vi "Process.vi"(8 "error in":errorcluster, 11 "DSP":refnum<class "DSP.lvclass">) -> (0 "error out":errorcluster, 3 "DSP out":refnum<class "DSP.lvclass">)   [LabVIEW 2016, in "DSP.lvclass"]
doc: "---------------------------------------------------------------\nJKI State Machine Objects™\nhttp://jki.net/state-machine-objects/\nCopyright (C) 2005-2015, JKI <info@jki.net>\nALL RIGHTS RESERVED"
uses:
  DSP.lvclass
  C:/Program Files (x86)/National Instruments/LabVIEW 2016/vi.lib/JKI/JKI SMO/SMO/SMO.lvclass
  <vilib>/JKI/JKI SMO/SMO/Typedefs/Parent Call--Enum.ctl
  Typedefs/PrivateEvents--DSP.RunCalculation.ctl
  Typedefs/LP_Config.ctl
  DSP.lockin/Typedefs/Lockin_Config.ctl
  Typedefs/FFT_Config.ctl
  <vilib>/Analysis/4window.llb/windowTd.ctl
  <vilib>/measure/maspectr.llb/Power Spectrum and PSD Export Mode.ctl
  <vilib>/JKI/JKI SMO/SMO/SMO.lvclass
  DSP.lockin/DSP.lockin.lvclass
  <vilib>/Analysis/NI_AALPro.lvlib
  <vilib>/measure/NI_MAPro.lvlib
  DSP.Filter/DSP.Filter.lvclass
panel:
  # "For instructions on how to use the JKI State Machine Objects, examples and video tutorials, visit:\nhttp://jki.net/state-machine-objects/\n\nJKI State Machine Objects™\nhttp://jki.net/state-machine-objects/\nCopyright (C) 2005-2015, JKI <info@jki.net>\nALL RIGHTS RESERVED"
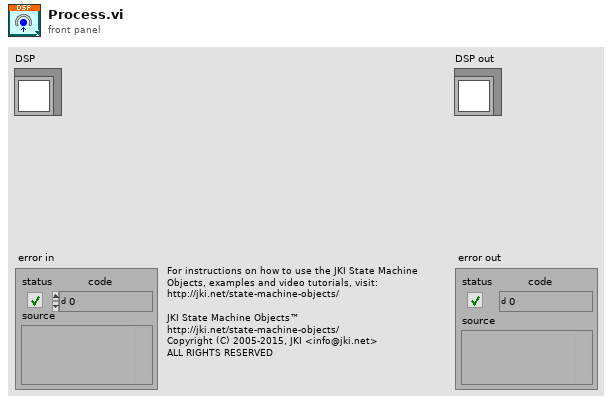
[diagram p1: front panel]
types:
  T1 = typedef "SMO.lvclass/Parent Call--Enum.ctl" = enum16{"Allows parent to run", "Does not request parent to run"}
  T2 = enum32{"invalid app kind", "Development System", "Run Time System", "Student Edition", "Embedded LabVIEW", "Evaluation", "Custom"}
  T3 = typedef "DSP.lvclass/PrivateEvents--DSP.RunCalculation.ctl" = cluster{"RunCalculation":cluster{"adjust gain":bool, "subtract offset":bool, "60 Hz prefilter":bool, "LP prefilter":bool, "lockin":bool, "FFT":bool, "gain":dbl[], "offset":dbl[], "LP config":T4, "Lockin config":T5, "FFT config":T6}}
  T4 = typedef "DSP.lvclass/LP_Config.ctl" = cluster{"high cutoff freq [Hz]":dbl}
  T5 = typedef "DSP.lockin.lvclass/Lockin_Config.ctl" = cluster{" f (Hz)":dbl, "phi (deg)":dbl, "TC (s)":dbl, "order":i32}[]
  T6 = typedef "DSP.lvclass/FFT_Config.ctl" = cluster{"averaging parameters":cluster{"averaging mode":enum16{"No averaging", "Vector averaging", "RMS averaging", "Peak hold"}, "weighting mode":enum16{"Linear", "Exponential"}, "number of averages":u32}, "window":T7, "export mode":T8, "window parameter":dbl, "restart averaging (F)":bool}
  T7 = typedef "NI_AALPro.lvlib/windowTd.ctl" = u32
  T8 = typedef "NI_MAPro.lvlib/Power Spectrum and PSD Export Mode.ctl" = u16
  T9 = enum32{"Invalid", "Standard", "Closed", "Hidden", "Minimized", "Maximized"}
  T10 = enum32{"Bad", "Idle", "Run top level", "Running"}
  T11 = typedef "DSP.lvclass/PrivateEvents--DSP.setWaveform.ctl" = waveform(dbl)[]
  T12 = cluster{"Core":cluster{"Current VI Reference":refnum<vi>, "Close Panel on Exit?":bool, "error":errorcluster}, "Self Reference":refnum<class "DSP.lvclass">, "Your string data":string, "Waveforms":waveform(dbl)[], "RunCalculation":cluster{"adjust gain":bool, "subtract offset":bool, "60 Hz prefilter":bool, "LP prefilter":bool, "lockin":bool, "FFT":bool, "gain":dbl[], "offset":dbl[], "LP config":T4, "Lockin config":T5, "FFT config":T6}}
  T13 = cluster{"adjust gain":bool, "subtract offset":bool, "60 Hz prefilter":bool, "LP prefilter":bool, "lockin":bool, "FFT":bool, "gain":dbl[], "offset":dbl[], "LP config":T4, "Lockin config":T5, "FFT config":T6}
  T14 = cluster{"Current VI Reference":refnum<vi>, "Close Panel on Exit?":bool, "error":errorcluster}
  T15 = typedef "SMO.lvclass/Protected Events.ctl" = cluster{"StopProcesses":refnum<user-event>, "AbortProcesses":refnum<user-event>, "Config Changed":refnum<user-event>, "Dependency":refnum<user-event>}
  T16 = typedef "DSP.lvclass/PrivateEvents--Cluster.ctl" = cluster{"setWaveform":refnum<user-event>, "RunCalculation":refnum<user-event>}
  T17 = typedef "DSP.lockin.lvclass/LockinResults.ctl" = T18[]
  T18 = typedef "DSP.lockin.lvclass/LockinResult.ctl" = cluster{"X":dbl, "Y":dbl, "R":dbl, "Theta":dbl, "AVG":dbl, "f":dbl}
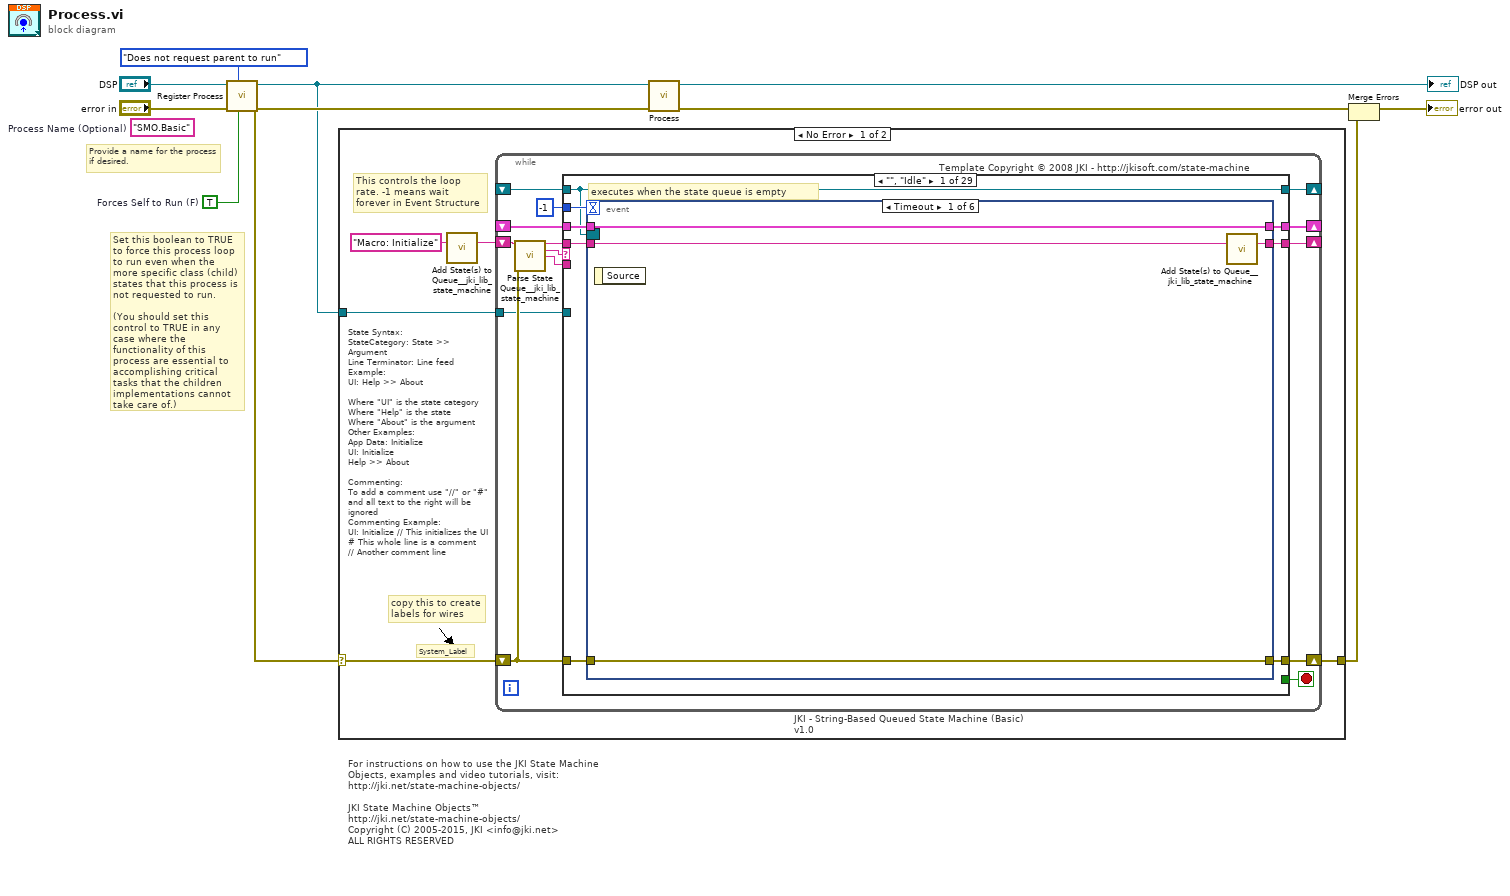
[diagram p0: block diagram]
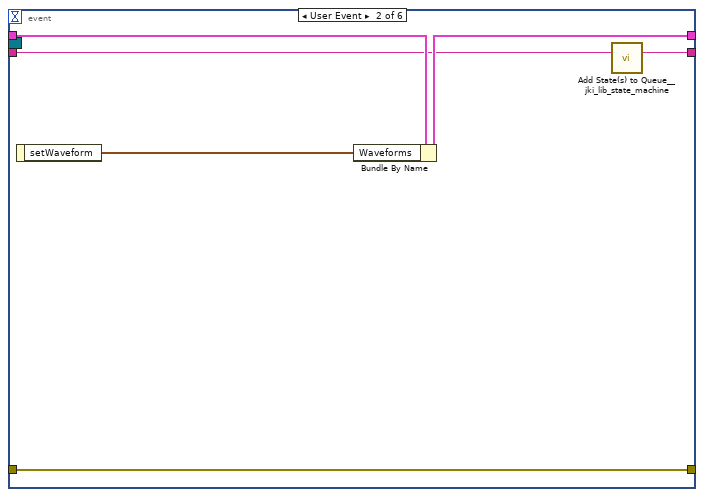
[diagram p2: hidden frame]
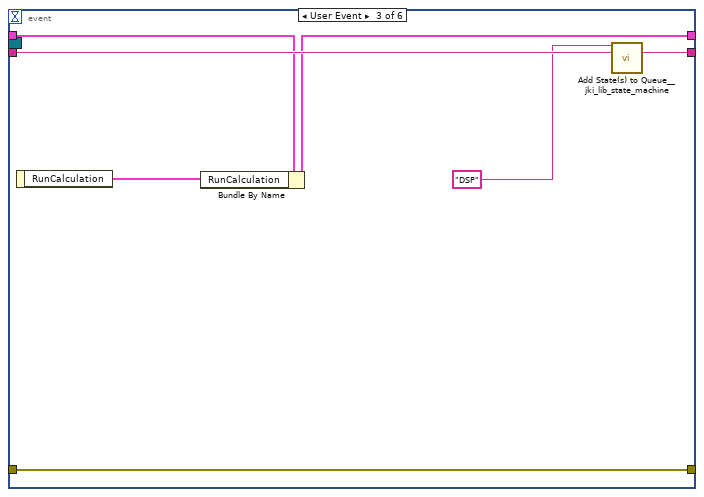
[diagram p3: hidden frame]
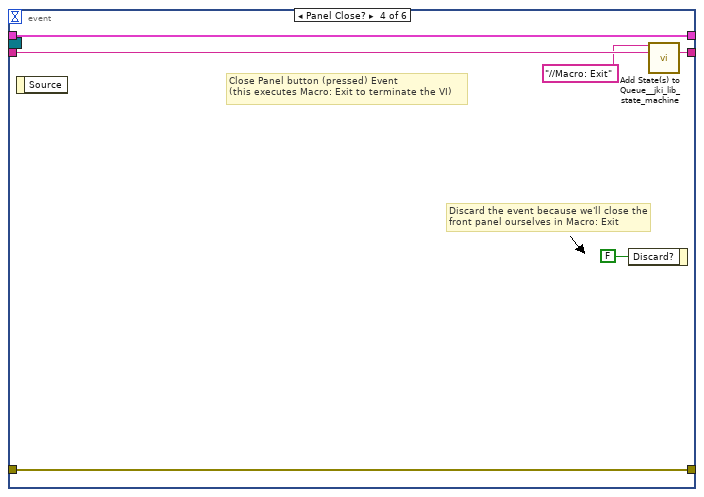
[diagram p4: hidden frame]
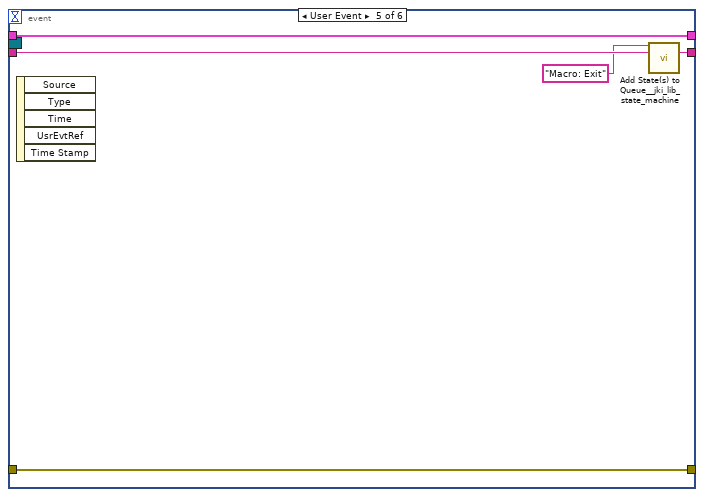
[diagram p5: hidden frame]
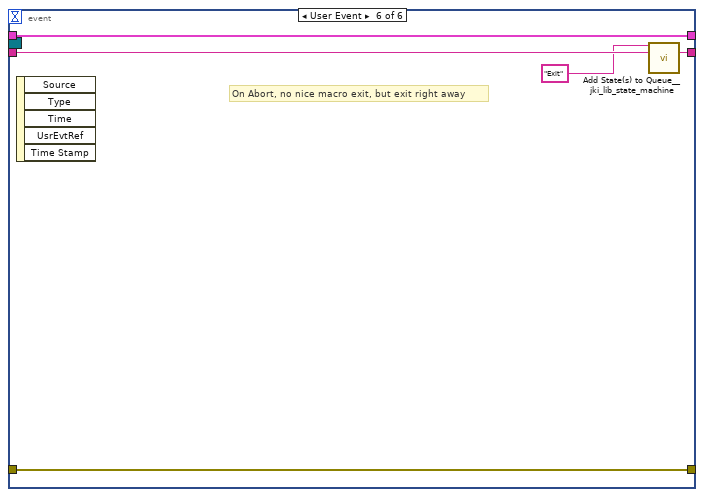
[diagram p6: hidden frame]
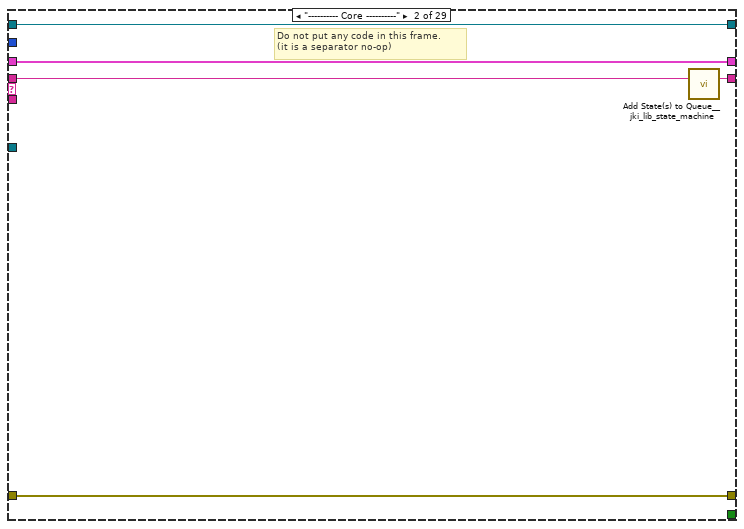
[diagram p7: hidden frame]
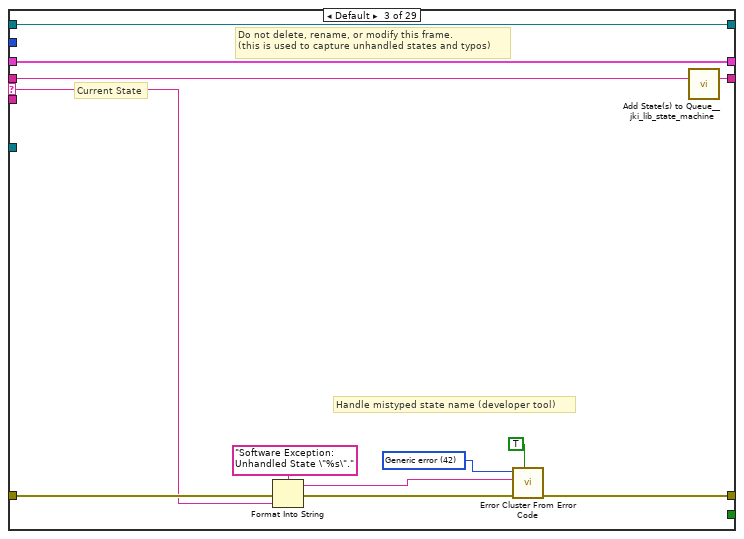
[diagram p8: hidden frame]
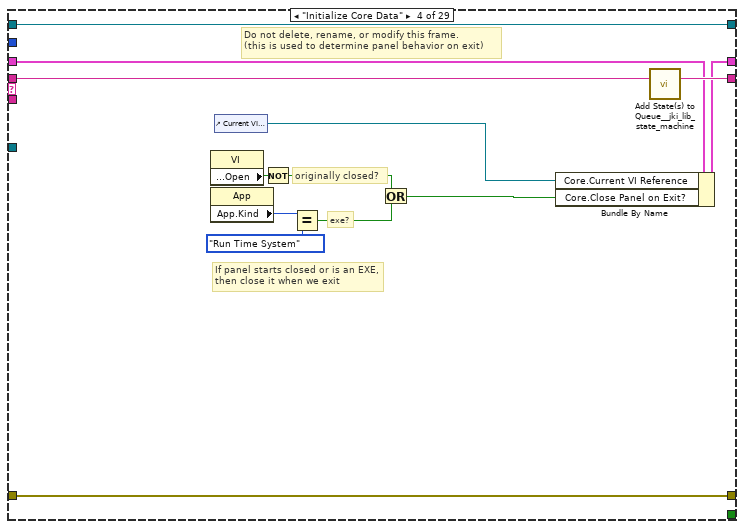
[diagram p9: hidden frame]
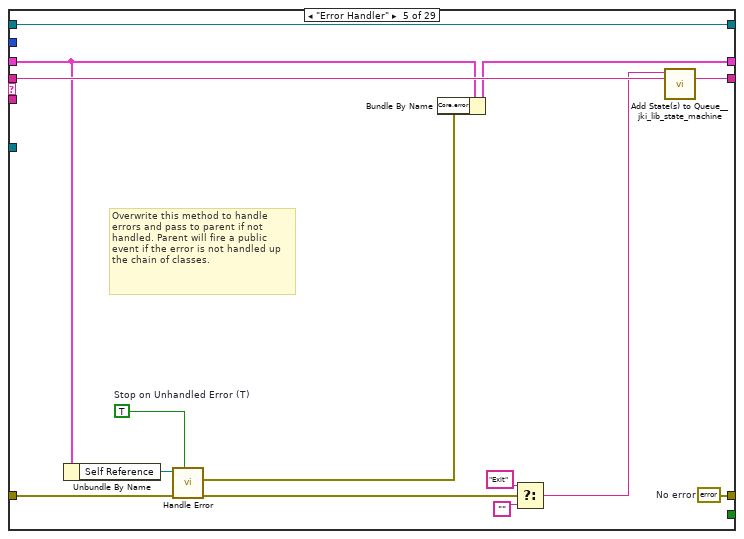
[diagram p10: hidden frame]
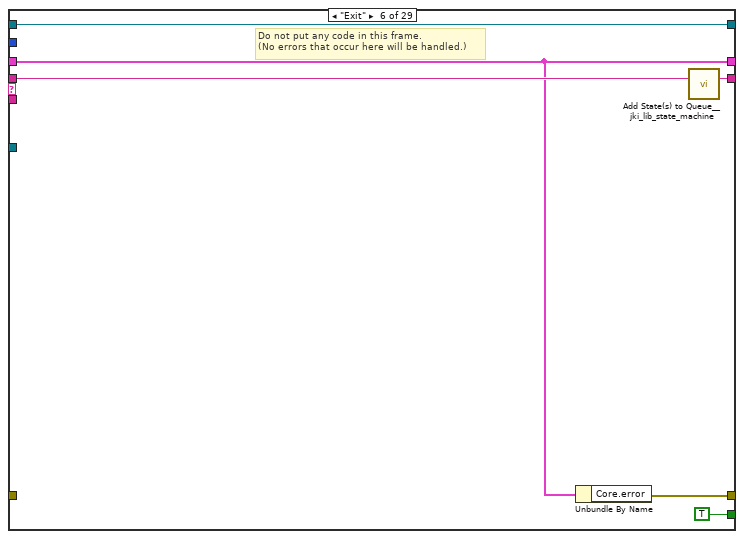
[diagram p11: hidden frame]
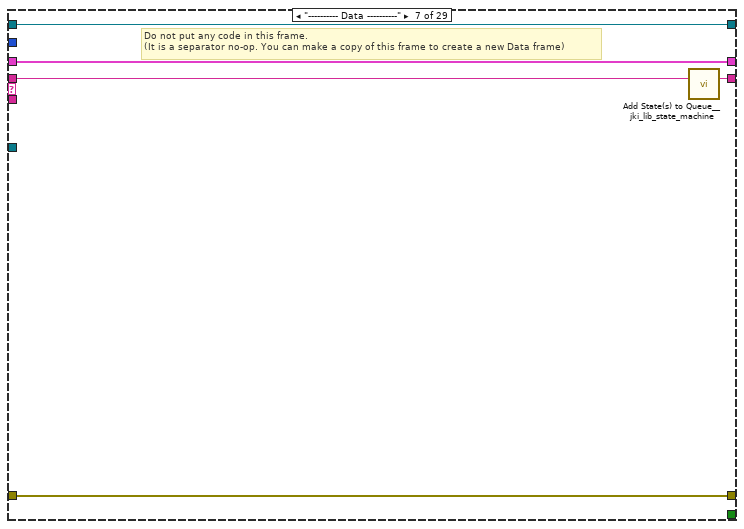
[diagram p12: hidden frame]
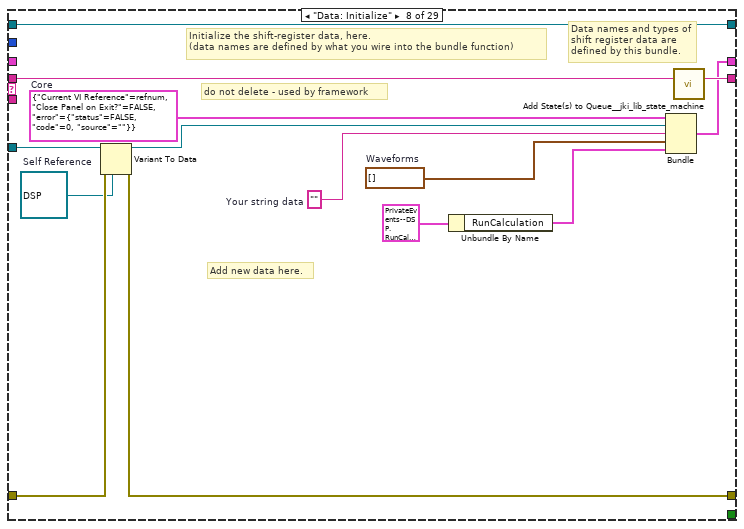
[diagram p13: hidden frame]
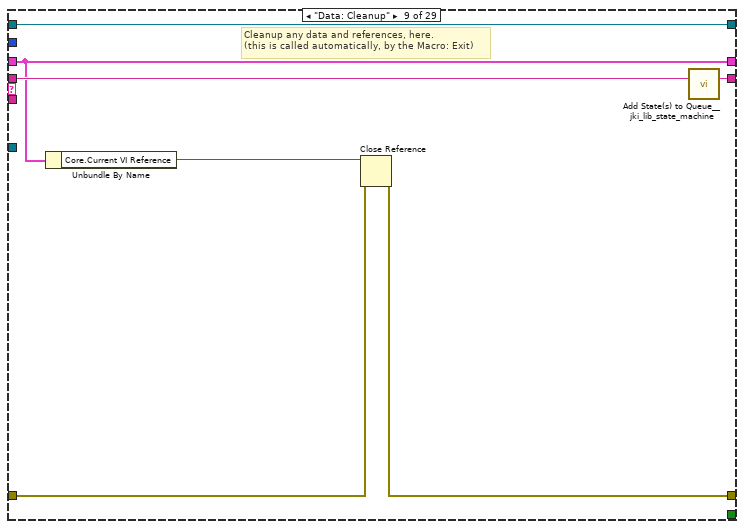
[diagram p14: hidden frame]
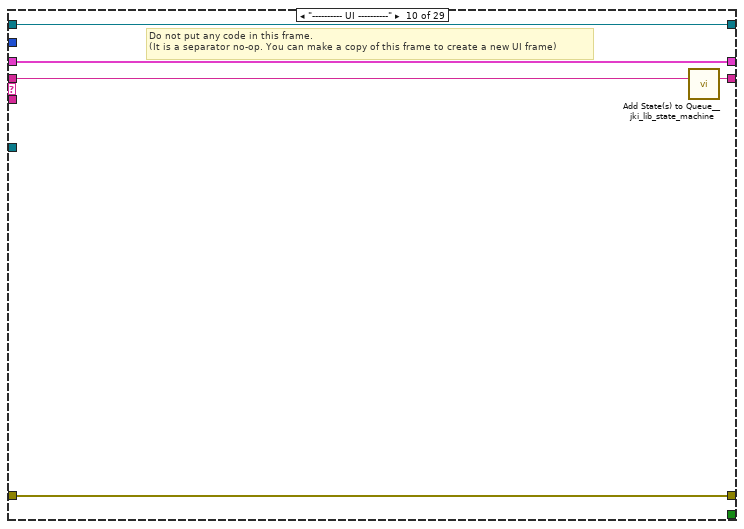
[diagram p15: hidden frame]
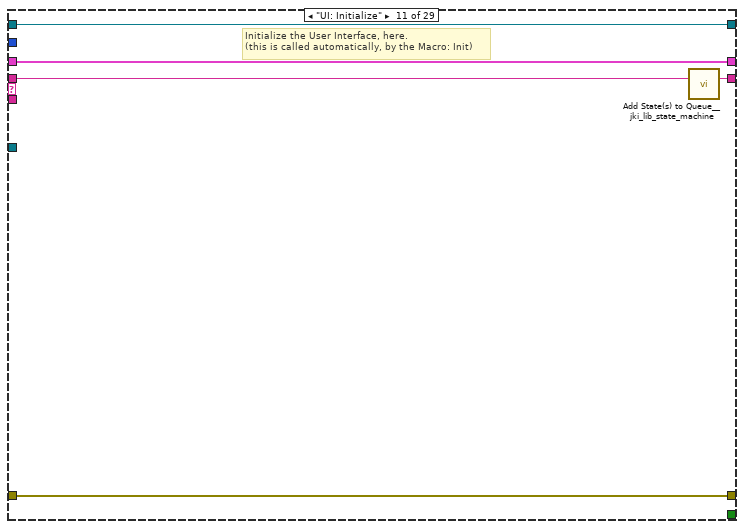
[diagram p16: hidden frame]
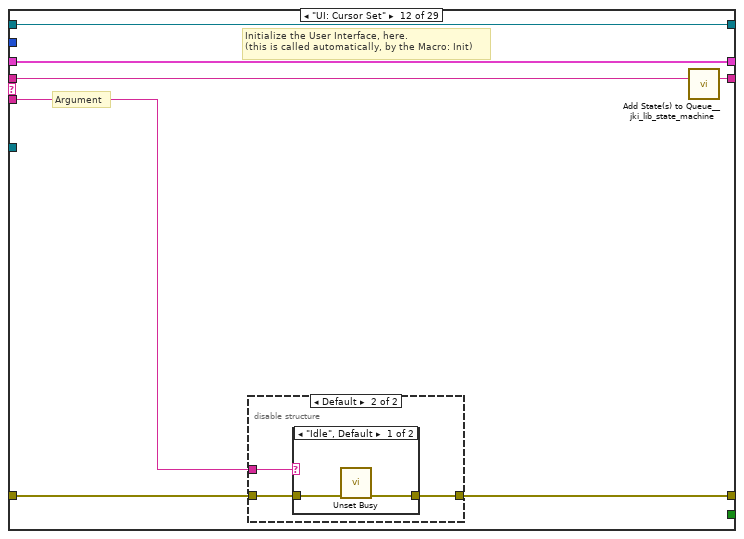
[diagram p17: hidden frame]
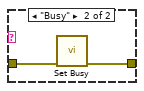
[diagram p19: hidden frame]
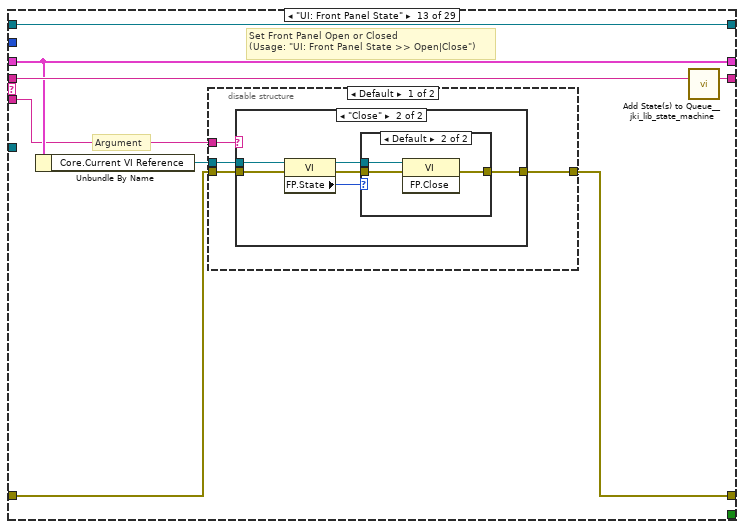
[diagram p20: hidden frame]
diagram:
  w1 = TRUE  # Forces Self to Run (F)
  (unwired) "SMO.Basic"  # Process Name (Optional)
  # "Provide a name for the process\nif desired."
  # "Set this boolean to TRUE to force this process loop to run even when the more specific class (child) states that this process is not requested to run.\n\n(You should set this control to TRUE in any case where the functionality of this process are essential to accomplishing critical tasks that the children implementations cannot take care of.)"
  # "For instructions on how to use the JKI State Machine Objects, examples and video tutorials, visit:\nhttp://jki.net/state-machine-objects/\n\nJKI State Machine Objects™\nhttp://jki.net/state-machine-objects/\nCopyright (C) 2005-2015, JKI <info@jki.net>\nALL RIGHTS RESERVED"
  n1 = call <vilib>:"Register Process.vi"("Forces Self to Run (F)"=w1, "Parent Call"=Parent_Call--Enum."Does not request parent to run", "error in (no error)"="error in", "SMO"="DSP") -> ("error out"=w7:errorcluster, "SMO out"=w6:refnum<class "DSP.lvclass">)  [unwired: 6 in]
  n2 = case shown="No Error" w7 {
    selector: w7 -> [w12 w368]
    tunnel: w6 -> [w13 _]
    tunnel: [w11 w368] -> w3
    frame No Error {
      # "State Syntax:\nStateCategory: State >> Argument\nLine Terminator: Line feed\nExample:\nUI: Help >> About\n\nWhere \"UI\" is the state category\nWhere \"Help\" is the state\nWhere \"About\" is the argument\nOther Examples:\nApp Data: Initialize\nUI: Initialize\nHelp >> About\n\nCommenting:\nTo add a comment use \"//\" or \"#\" and all text to the right will be ignored\nCommenting Example:\nUI: Initialize // This initializes the UI\n# This whole line is a comment\n// Another comment line"
      # "copy this to create labels for wires"
      # "This controls the loop rate. -1 means wait forever in Event Structure"
      # "System_Label"
      n3 = call <vilib>:"Add State(s) to Queue__jki_lib_state_machine.vi"("State(s) in (\"\")"="Macro: Initialize") -> ("States Out"=w15:string)  [unwired: 14 in]
      n4 = while "JKI - String-Based Queued State Machine (Basic) v1.0" {
        shift-right: [w22] -> _
        shift-left: _ -> [w21]
        shift-right: [w25] -> w11
        shift-left: w12 -> [w19]
        shift-right: [w24] -> _
        shift-left: w15 -> [w26]
        tunnel: w13 -> [w18]
        shift-right: [w17] -> _
        shift-left: _ -> [w16]
        stop <- w23 stop-if-true
        # "Template Copyright © 2008 JKI - http://jkisoft.com/state-machine"
        n5 = call <vilib>:"Parse State Queue__jki_lib_state_machine.vi"("State Queue"=w26, "Error In (no error)"=w19) -> ("Remaining States"=w28:string, "Current State"=w29:string, "Arguments"=w27:string)  [unwired: 11 in]
        n6 = case shown="\"\", \"Idle\"" w29 {
          selector: w29 -> [_ _ w77 _ _ _ _ _ _ _ _ _ _ _ _ _ _ _ _ _ _ _ _ _ _ _ _ _ _]
          tunnel: w28 -> [w37 w75 w81 w100 w114 w120 w125 w139 w146 w151 w156 w163 w179 w211 w225 w239 w244 w255 w260 w273 w279 w284 w310 w319 w328 w337 w347 w358 w367]
          tunnel: w27 -> [_ _ _ _ _ _ _ _ _ _ _ w157 w173 _ _ _ _ _ _ _ _ _ _ _ _ _ _ _ _]
          tunnel: w21 -> [w35 w72 w79 w91 w108 w116 w122 _ w141 w148 w154 w161 w175 w208 w221 w230 w241 w252 w257 w271 w277 w282 w306 w315 w324 w334 w344 w355 w363]
          tunnel: [w34 w73 w83 w97 w109 w115 w123 w134 w142 w149 w153 w158 w176 w209 w223 w237 w242 w246 w258 w266 w275 w280 w307 w316 w325 w329 w338 w348 w364] -> w25
          tunnel: w19 -> [w33 w73 w82 w97 w110 _ w123 w135 w143 w149 w153 w159 w177 w209 w223 w237 w242 w247 w258 w267 w275 w280 w307 w316 w325 w330 w339 w354 w364]
          tunnel: [w36 w74 w80 w99 w113 w119 w124 w138 w145 w150 w155 w162 w178 w210 w224 w238 w243 w254 w259 w272 w278 w283 w309 w318 w327 w336 w346 w357 w366] -> w24
          tunnel: [_ _ _ _ _ TRUE _ _ _ _ _ _ _ _ _ _ _ _ _ _ _ _ _ _ _ _ _ _ _] -> w23
          tunnel: [w32 w72 w79 w98 w107 w116 w122 w137 w141 w148 w154 w161 w175 w208 w221 w230 w241 w252 w257 w271 w277 w282 w306 w314 w323 w333 w343 w355 w362] -> w22
          tunnel: -1 ("Timeout") -> [w31 _ _ _ _ _ _ _ _ _ _ _ _ _ _ _ _ _ _ _ _ _ _ _ _ _ _ _ _]
          tunnel: w18 -> [_ _ _ _ _ _ _ w132 _ _ _ _ _ _ _ _ _ _ _ _ _ _ _ _ _ _ _ _ _]
          tunnel: [w30 w71 w76 w88 w112 w117 w121 w130 w140 w147 w152 w160 w172 w207 w222 w231 w240 w253 w256 w270 w276 w281 w308 w317 w326 w335 w345 w356 w365] -> w17
          tunnel: w16 -> [w30 w71 w76 w88 w112 w117 w121 w130 w140 w147 w152 w160 w172 w207 w222 w231 w240 w253 w256 _ w276 w281 w308 w317 w326 w335 w345 w356 w365]
          frame "", "Idle" {
            # "executes when the state queue is empty"
            n7 = event shown="[0] Timeout" {
              selector: w30 -> [_ _ _ _ _ _]
              dyn-events: _ -> [_ _ _ _ _ _]
              timeout: w31 -> [_ _ _ _ _ _]
              tunnel: w37 -> [w41 w43 w53 w60 w65 w70]
              tunnel: [w40 w42 w52 w59 w64 w69] -> w36
              tunnel: w35 -> [w39 w47 w51 w57 w62 w67]
              tunnel: [w38 w44 w54 w58 w63 w68] -> w34
              tunnel: w33 -> [w38 w44 w54 w58 w63 w68]
              tunnel: [w39 w45 w49 w57 w62 w67] -> w32
              event Timeout {
                n8 = event-data() -> ()  [unwired: 1 in, 1 out]
                n9 = call <vilib>:"Add State(s) to Queue__jki_lib_state_machine.vi"("State(s) in (\"\")"=w41) -> ("States Out"=w40:string)  [unwired: 14 in]
              }
              event User Event {
                n10 = event-data() -> ("setWaveform"=w46:T11)  [unwired: 1 in]
                n11 = Bundle By Name(cluster=w47, "Waveforms"=w46) -> (w45:T12)
                n12 = call <vilib>:"Add State(s) to Queue__jki_lib_state_machine.vi"("State(s) in (\"\")"=w43) -> ("States Out"=w42:string)  [unwired: 14 in]
              }
              event User Event {
                n13 = event-data() -> ("RunCalculation"=w50:T13)  [unwired: 1 in]
                n14 = Bundle By Name(cluster=w51, "RunCalculation"=w50) -> (w49:T12)
                n15 = call <vilib>:"Add State(s) to Queue__jki_lib_state_machine.vi"("State(s) in Front (\"\")"="DSP" ("State(s) in Front (\"\")"), "State(s) in (\"\")"=w53) -> ("States Out"=w52:string)  [unwired: 13 in]
              }
              event Panel Close? {
                # "Discard the event because we'll close the front panel ourselves in Macro: Exit"
                # "Close Panel button (pressed) Event\n(this executes Macro: Exit to terminate the VI)"
                n16 = event-data() -> ()  [unwired: 1 in, 1 out]
                n17 = event-data("Discard?"=FALSE) -> ()  [unwired: 1 in, 1 out]
                n18 = call <vilib>:"Add State(s) to Queue__jki_lib_state_machine.vi"("State(s) in Front (\"\")"="//Macro: Exit", "State(s) in (\"\")"=w60) -> ("States Out"=w59:string)  [unwired: 13 in]
              }
              event User Event {
                n19 = event-data() -> ()  [unwired: 1 in, 5 out]
                n20 = call <vilib>:"Add State(s) to Queue__jki_lib_state_machine.vi"("State(s) in Front (\"\")"="Macro: Exit", "State(s) in (\"\")"=w65) -> ("States Out"=w64:string)  [unwired: 13 in]
              }
              event User Event {
                # "On Abort, no nice macro exit, but exit right away"
                n21 = event-data() -> ()  [unwired: 1 in, 5 out]
                n22 = call <vilib>:"Add State(s) to Queue__jki_lib_state_machine.vi"("State(s) in Front (\"\")"="Exit", "State(s) in (\"\")"=w70) -> ("States Out"=w69:string)  [unwired: 13 in]
              }
            }
          }
          frame "---------- Core ----------" {
            # "Do not put any code in this frame.\n(it is a separator no-op)"
            n23 = call <vilib>:"Add State(s) to Queue__jki_lib_state_machine.vi"("State(s) in (\"\")"=w75) -> ("States Out"=w74:string)  [unwired: 14 in]
          }
          frame Default {
            w86 = 42 items=["No error", "Argument error", "Memory is full", "Out of zone", "End of file", "File already open", "Generic file I/O error", "File not found", "File permission error", "Disk is full", "Duplicate path", "Too many files open", "System feature not enabled", "Resource file not found", "Cannot add resource", "Resource not found", "Image not found", "Image memory error", "Pen does not exist", "Config type invalid", "Config token not found", "Config parse error", "Config memory error", "Bad external code format", "Bad external code offset", "External code not present", "Null window", "Destroy window error", "Null menu", "Print aborted", "Bad print record", "Print driver error", "Windows error during printing", "Memory error during printing", "Print dialog error", "Generic print error", "Invalid device refnum", "Device not found", "Device parameter error", "Device unit error", "Cannot open device", "Device call aborted", "Generic error", "Cancelled by user", "Object ID too low", "Object ID too high", "Object not in heap", "Unknown heap", "Unknown object (invalid DefProc)", "Unknown object (DefProc not in table)", "Message out of range", "Invalid (null) method", "Unknown message", "Manager call not supported", "Bad address", "Network operation in progress", "Network operation timed out", "Connection is busy", "Network attribute not supported", "Network error", "Address in use", "System out of memory", "Connection aborted", "Connection refused", "Not connected", "Already connected", "Connection closed", "Initialization error (interapplication manager)", "Bad occurrence", "Wait on unbound occurrence handler", "Occurrence queue overflow", "Datalog type conflict", "Unused", "Unrecognized type (interapplication manager)", "Memory corrupt", "Failed to make temporary DLL", "Old CIN version", "Drag socket not found", "Failed to load drop-object", "Failed to register OLE object", "Failed to release OLE object", "Format specifier type mismatch", "Unknown format specifier", "Too few format specifiers", "Too many format specifiers", "Scan failed", "Newer CIN version", "Error converting to variant", "Runtime menu error", "Password tampered", "Variant attribute not found", "Incompatible variant data type", "Event data is not available", "Event Store is not present", "Occurrence is not found", "Event Queue is not created", "Event info is not available", "Refnum passed is NULL", "Error retrieving Class GUID", "Error retrieving CoClass GUID", "Error retrieving TypeLib GUID.", "Bad built application magic bytes.", "Specific driver is different from the specific driver associated with the Logical Name.", "There is no session opened to the class driver.", "Max Error", "MAX - Error with config objects", "MAX - Error loading configuration", "MAX - Group not supported"]
            # "Current State"
            # "Do not delete, rename, or modify this frame.\n(this is used to capture unhandled states and typos)"
            # "Handle mistyped state name (developer tool)"
            n24 = Format Into String(format string="Software Exception: Unhandled State \"%s\"." ("message"), error in=w82, w77) -> (resulting string=w85:string, error out=w84:errorcluster)  [unwired: 1 in]
            n25 = call <vilib>:"Error Cluster From Error Code.vi"("show call chain? (False)"=TRUE, "error in (no error)"=w84, "error message (\"\")"=w85, "error code (0)"=w86) -> ("error out"=w83:errorcluster)  [unwired: 5 in]
            n26 = call <vilib>:"Add State(s) to Queue__jki_lib_state_machine.vi"("State(s) in (\"\")"=w81) -> ("States Out"=w80:string)  [unwired: 14 in]
          }
          frame "Initialize Core Data" {
            # "Do not delete, rename, or modify this frame.\n(this is used to determine panel behavior on exit)"
            # "originally closed?"
            # "exe?"
            # "If panel starts closed or is an EXE, then close it when we exit"
            n27 = property class="VI"() -> ("Front Panel.Open"=w96:bool)  [unwired: 2 in, 2 out]
            n28 = property class="App"() -> ("App.Kind"=w95:T2)  [unwired: 2 in, 2 out]
            n29 = control-ref of="Current VI Reference"() -> (w89:refnum<vi>)
            n30 = Not(x=w96) -> (.not. x?=w93:bool)
            n31 = Equal?(x=w95, y=T2."Run Time System" ("Application:Kind")) -> (x = y?=w92:bool)
            n32 = Or(x=w93, y=w92) -> (x .or. y?=w90:bool)
            n33 = Bundle By Name(cluster=w91, "Core.Current VI Reference"=w89, "Core.Close Panel on Exit?"=w90) -> (w98:T12)
            n34 = call <vilib>:"Add State(s) to Queue__jki_lib_state_machine.vi"("State(s) in (\"\")"=w100) -> ("States Out"=w99:string)  [unwired: 14 in]
          }
          frame "Error Handler" {
            w101 = TRUE  # Stop on Unhandled Error (T)
            w109 = errorcluster {"status"=FALSE, "code"=0, "source"=""}  # No error
            # "Overwrite this method to handle errors and pass to parent if not handled. Parent will fire a public event if the error is not handled up the chain of classes."
            n35 = Unbundle By Name(w108) -> ("Self Reference"=w111:refnum<class "DSP.lvclass">)
            n36 = call-dynamic "Handle Error.vi"("Stop on Unhandled Error (T)"=w101, "error in"=w110, "SMO"=w111) -> ("handling error"=w102:errorcluster, "Unhandled error"=w105:errorcluster)  [unwired: 6 in, 1 out]
            n37 = Bundle By Name(cluster=w108, "Core.error"=w105) -> (w107:T12)
            n38 = Select(t="Exit", s=w102, f="") -> (s? t:f=w106:string)
            n39 = call <vilib>:"Add State(s) to Queue__jki_lib_state_machine.vi"("State(s) in Front (\"\")"=w106, "State(s) in (\"\")"=w114) -> ("States Out"=w113:string)  [unwired: 13 in]
          }
          frame "Exit" {
            # "Do not put any code in this frame.\n(No errors that occur here will be handled.)"
            n40 = Unbundle By Name(w116) -> ("Core.error"=w115:errorcluster)
            n41 = call <vilib>:"Add State(s) to Queue__jki_lib_state_machine.vi"("State(s) in (\"\")"=w120) -> ("States Out"=w119:string)  [unwired: 14 in]
          }
          frame "---------- Data ----------" {
            # "Do not put any code in this frame.\n(It is a separator no-op. You can make a copy of this frame to create a new Data frame)"
            n42 = call <vilib>:"Add State(s) to Queue__jki_lib_state_machine.vi"("State(s) in (\"\")"=w125) -> ("States Out"=w124:string)  [unwired: 14 in]
          }
          frame "Data: Initialize" {
            w128 = waveform(dbl)[] []  # Waveforms
            w129 = T14 {"Current VI Reference"=refnum, "Close Panel on Exit?"=FALSE, "error"={"status"=FALSE, "code"=0, "source"=""}}  # Core
            w133 = refnum<class "DSP.lvclass"> refnum  # Self Reference
            w136 = ""  # Your string data
            # "do not delete - used by framework"
            # "Add new data here."
            # "Data names and types of shift register data are defined by this bundle."
            # "Initialize the shift-register data, here.\n(data names are defined by what you wire into the bundle function)"
            n43 = Variant To Data(error in=w135, type=w133, Variant=w132) -> (data=w131:refnum<class "DSP.lvclass">, error out=w134:errorcluster)
            n44 = Unbundle By Name(T3 {"RunCalculation"={"adjust gain"=FALSE, "subtract offset"=FALSE, "60 Hz prefilter"=FALSE, "LP prefilter"=FALSE, "lockin"=FALSE, "FFT"=FALSE, "gain"=[], "offset"=[], "LP config"={"high cutoff freq [Hz]"=0.45}, "Lockin config"=[], "FFT config"={"averaging parameters"={"averaging mode"=enum."RMS averaging", "weighting mode"=enum."Exponential", "number of averages"=10}, "window"=1, "export mode"=0, "window parameter"=nan, "restart averaging (F)"=FALSE}}} ("RunCalculation")) -> ("RunCalculation"=w126:T13)
            n45 = Bundle("Core"=w129, "Self Reference"=w131, "Your string data"=w136, "Waveforms"=w128, "RunCalculation"=w126) -> (w137:T12)  [unwired: 1 in]
            n46 = call <vilib>:"Add State(s) to Queue__jki_lib_state_machine.vi"("State(s) in (\"\")"=w139) -> ("States Out"=w138:string)  [unwired: 14 in]
          }
          frame "Data: Cleanup" {
            # "Cleanup any data and references, here.\n(this is called automatically, by the Macro: Exit)"
            n47 = Unbundle By Name(w141) -> ("Core.Current VI Reference"=w144:refnum<vi>)
            n48 = Close Reference(reference=w144, error in (no error)=w143) -> (error out=w142:errorcluster)
            n49 = call <vilib>:"Add State(s) to Queue__jki_lib_state_machine.vi"("State(s) in (\"\")"=w146) -> ("States Out"=w145:string)  [unwired: 14 in]
          }
          frame "---------- UI ----------" {
            # "Do not put any code in this frame.\n(It is a separator no-op. You can make a copy of this frame to create a new UI frame)"
            n50 = call <vilib>:"Add State(s) to Queue__jki_lib_state_machine.vi"("State(s) in (\"\")"=w151) -> ("States Out"=w150:string)  [unwired: 14 in]
          }
          frame "UI: Initialize" {
            # "Initialize the User Interface, here.\n(this is called automatically, by the Macro: Init)"
            n51 = call <vilib>:"Add State(s) to Queue__jki_lib_state_machine.vi"("State(s) in (\"\")"=w156) -> ("States Out"=w155:string)  [unwired: 14 in]
          }
          frame "UI: Cursor Set" {
            # "Argument"
            # "Initialize the User Interface, here.\n(this is called automatically, by the Macro: Init)"
            n52 = disable-structure shown="Default" {
              disable-tunnel: w159 -> [w164 w167]
              disable-tunnel: [w164 w166] -> w158
              disable-tunnel: w157 -> [_ w165]
              frame condition #0 {
              }
              frame condition #1 (active) {
                n53 = case shown="\"Idle\", Default" w165 {
                  tunnel: w167 -> [w169 w171]
                  tunnel: [w168 w170] -> w166
                  frame "Idle", Default {
                    n54 = call <vilib>:"Unset Busy.vi"("error in (no error)"=w169) -> ("error out"=w168:errorcluster)  [unwired: 10 in]
                  }
                  frame "Busy" {
                    n55 = call <vilib>:"Set Busy.vi"("error in (no error)"=w171) -> ("error out"=w170:errorcluster)  [unwired: 9 in, 1 out]
                  }
                }
              }
            }
            n56 = call <vilib>:"Add State(s) to Queue__jki_lib_state_machine.vi"("State(s) in (\"\")"=w163) -> ("States Out"=w162:string)  [unwired: 14 in]
          }
          frame "UI: Front Panel State" {
            # "Argument"
            # "Set Front Panel Open or Closed\n(Usage: \"UI: Front Panel State >> Open|Close\")"
            n57 = Unbundle By Name(w175) -> ("Core.Current VI Reference"=w174:refnum<vi>)
            n58 = disable-structure shown="Default" {
              disable-tunnel: w177 -> [w183 w206]
              disable-tunnel: [w182 w206] -> w176
              disable-tunnel: w174 -> [w181 _]
              disable-tunnel: w173 -> [w180 _]
              frame condition #0 (active) {
                n59 = case shown="\"Close\"" w180 {
                  tunnel: w183 -> [w187 w200]
                  tunnel: [w189 w201] -> w182
                  tunnel: w181 -> [w188 w198]
                  frame "Open", Default {
                    n60 = property class="VI"(reference=w188, error in=w187) -> (reference out=w185:refnum<vi>, error out=w186:errorcluster, "FP.State"=w184:T9)
                    n61 = case shown="\"Closed\"" w184 {
                      tunnel: [w192 w195] -> w189
                      tunnel: w186 -> [w191 w195]
                      tunnel: w185 -> [w190 _]
                      frame "Closed" {
                        n62 = invoke class="VI" method="FP.Open"(reference=w190, error in=w191, "Activate"=TRUE, "State"=T9."Standard") -> (error out=w192:errorcluster)  [unwired: 1 in, 4 out]
                      }
                      frame Default {
                      }
                    }
                  }
                  frame "Close" {
                    n63 = property class="VI"(reference=w198, error in=w200) -> (reference out=w197:refnum<vi>, error out=w199:errorcluster, "FP.State"=w196:T9)
                    n64 = case shown="Default" w196 {
                      tunnel: [w202 w205] -> w201
                      tunnel: w199 -> [w202 w204]
                      tunnel: w197 -> [_ w203]
                      frame "Invalid", "Closed" {
                      }
                      frame Default {
                        n65 = invoke class="VI" method="FP.Close"(reference=w203, error in=w204) -> (error out=w205:errorcluster)  [unwired: 1 in, 2 out]
                      }
                    }
                  }
                }
              }
              frame condition #1 {
              }
            }
            n66 = call <vilib>:"Add State(s) to Queue__jki_lib_state_machine.vi"("State(s) in (\"\")"=w179) -> ("States Out"=w178:string)  [unwired: 14 in]
          }
          frame "---------- Macro ----------" {
            # "Do not put any code in this frame.\n(It is a separator no-op. You can make a copy of this frame to create a new Macro frame)"
            n67 = call <vilib>:"Add State(s) to Queue__jki_lib_state_machine.vi"("State(s) in (\"\")"=w211) -> ("States Out"=w210:string)  [unwired: 14 in]
          }
          frame "Macro: Initialize" {
            w216 = "//UI: Initialize\n//UI: Front Panel State >> Open"  # //UI: Initialize //UI: Front Panel State >> Open
            w212 = "Process: Sync"
            # "Initialization Macro\n(This is called once, when the VI starts)"
            n68 = control-ref of="This VI"() -> (w214:refnum<vi>)
            n69 = property class="VI"(reference=w214) -> ("Exec.State"=w213:T10)  [unwired: 1 in, 2 out]
            n70 = Equal?(x=w213, y=T10."Run top level") -> (x = y?=w219:bool)
            n71 = Select(t=w212, s=w219, f="") -> ()  [unwired: 1 out]
            n72 = call <vilib>:"Add State(s) to Queue__jki_lib_state_machine.vi"("State(s) in Front (\"\")"="Data: Initialize\nInitialize Core Data\nEvents: Register", "State(s) in (\"\")"=w212, "State(s) at Back (\"\")"=w216) -> ("States Out"=w215:string)  [unwired: 12 in]
            n73 = call <vilib>:"Add State(s) to Queue__jki_lib_state_machine.vi"("State(s) in Front (\"\")"=w215, "State(s) in (\"\")"=w225) -> ("States Out"=w224:string)  [unwired: 13 in]
          }
          frame "Macro: Exit" {
            # "Exit Macro\n(This is called once, when the VI exits)"
            n74 = Unbundle By Name(w230) -> ("Core.Close Panel on Exit?"=w236:bool)
            n75 = Select(t="UI: Front Panel State >> Close", s=w236, f="") -> (s? t:f=w233:string)
            n76 = call <vilib>:"Add State(s) to Queue__jki_lib_state_machine.vi"("State(s) in Front (\"\")"="Data: Cleanup\nEvents: Unregister", "State(s) in (\"\")"="Process: Sync", "State(s) at Back (\"\")"="Exit") -> ("States Out"=w227:string)  [unwired: 12 in]
            n77 = call <vilib>:"Add State(s) to Queue__jki_lib_state_machine.vi"("State(s) in (\"\")"=w233, "State(s) at Back (\"\")"=w227) -> ("States Out"=w232:string)  [unwired: 13 in]
            n78 = call <vilib>:"Add State(s) to Queue__jki_lib_state_machine.vi"("State(s) in Front (\"\")"=w232, "State(s) in (\"\")"=w239) -> ("States Out"=w238:string)  [unwired: 13 in]
          }
          frame "---------- Process ----------" {
            # "Template Separator\n(You can make a copy of, or modify, this frame)"
            n79 = call <vilib>:"Add State(s) to Queue__jki_lib_state_machine.vi"("State(s) in (\"\")"=w244) -> ("States Out"=w243:string)  [unwired: 14 in]
          }
          frame "Process: Sync" {
            n80 = Unbundle By Name(w252) -> ("Self Reference"=w248:refnum<class "DSP.lvclass">)
            n81 = call <vilib>:"WaitOnProcessSync.vi"("error in (no error)"=w247, "SMO"=w248) -> ("error out"=w246:errorcluster, "Don't run?"=w251:bool)  [unwired: 7 in, 1 out]
            n82 = Select(t="Data: Cleanup\nEvents: Unregister\nExit", s=w251, f="") -> (s? t:f=w245:string)
            n83 = call <vilib>:"Add State(s) to Queue__jki_lib_state_machine.vi"("State(s) in Front (\"\")"=w245, "State(s) in (\"\")"=w255) -> ("States Out"=w254:string)  [unwired: 13 in]
          }
          frame "---------- Events ----------" {
            # "Template Separator\n(You can make a copy of, or modify, this frame)"
            n84 = call <vilib>:"Add State(s) to Queue__jki_lib_state_machine.vi"("State(s) in (\"\")"=w260) -> ("States Out"=w259:string)  [unwired: 14 in]
          }
          frame "Events: Register" {
            # "Expand to add\nmore events"
            n85 = Unbundle By Name(w271) -> ("Self Reference"=w268:refnum<class "DSP.lvclass">)
            n86 = call <vilib>:"GetProtectedEvents.vi"("SMO"=w268) -> ("error out"=w262:errorcluster, "SMO Protected Events"=w269:T15, "SMO out"=w264:refnum<class "DSP.lvclass">)  [unwired: 8 in]
            n87 = call "DSP.GetPrivateEvents.vi"("error in (no error)"=w262, "DSP"=w264) -> ("error out"=w261:errorcluster, "Private Events"=w263:T16)  [unwired: 7 in, 1 out]
            n88 = register-events(w269, w263) -> (reference out=w270:refnum<event-registration>, error out=w265:errorcluster)  [unwired: 2 in]
            n89 = Merge Errors(w267, w265, w261) -> (w266:errorcluster)
            n90 = call <vilib>:"Add State(s) to Queue__jki_lib_state_machine.vi"("State(s) in (\"\")"=w273) -> ("States Out"=w272:string)  [unwired: 14 in]
          }
          frame "Events: Unregister" {
            n91 = Unregister For Events(event registration refnum=w276, error in=w275) -> (error out=w274:errorcluster)
            n92 = call <vilib>:"Clear Errors.vi"("error in (no error)"=w274) -> ()  [unwired: 5 in, 2 out]
            n93 = call <vilib>:"Add State(s) to Queue__jki_lib_state_machine.vi"("State(s) in (\"\")"=w279) -> ("States Out"=w278:string)  [unwired: 14 in]
          }
          frame "---------- Action ----------" {
            n94 = call <vilib>:"Add State(s) to Queue__jki_lib_state_machine.vi"("State(s) in (\"\")"=w284) -> ("States Out"=w283:string)  [unwired: 14 in]
          }
          frame "DSP" {
            w286 = "\n"
            w293 = "" ("f")
            # "decision tree queues other states"
            n95 = Unbundle By Name(w306) -> ("RunCalculation.adjust gain"=w305:bool, "RunCalculation.subtract offset"=w304:bool, "RunCalculation.60 Hz prefilter"=w303:bool, "RunCalculation.LP prefilter"=w302:bool, "RunCalculation.lockin"=w301:bool, "RunCalculation.FFT"=w300:bool)
            n96 = Select(t="DSP: Gain" ("State(s) in Front (\"\")"), s=w305, f=w293) -> (s? t:f=w292:string)
            n97 = Select(t="DSP: Offset" ("State(s) in Front (\"\")"), s=w304, f=w293) -> (s? t:f=w291:string)
            n98 = Select(t="DSP: 60Hz Filter" ("State(s) in Front (\"\")"), s=w303, f=w293) -> (s? t:f=w290:string)
            n99 = Select(t="DSP: LP Filter" ("State(s) in Front (\"\")"), s=w302, f=w293) -> (s? t:f=w289:string)
            n100 = Select(t="DSP: Lockin" ("State(s) in Front (\"\")"), s=w301, f=w293) -> (s? t:f=w288:string)
            n101 = Select(t="DSP: FFT" ("State(s) in Front (\"\")"), s=w300, f=w293) -> (s? t:f=w285:string)
            n102 = Concatenate Strings(w292, w286, w291, w286, w290, w286, w289, w286, w288, w286, w285) -> (w287:string)
            n103 = call <vilib>:"Add State(s) to Queue__jki_lib_state_machine.vi"("State(s) in Front (\"\")"=w287, "State(s) in (\"\")"=w310) -> ("States Out"=w309:string)  [unwired: 13 in]
          }
          frame "DSP: Gain" {
            # "Divide by amplifier gain"
            n104 = Unbundle By Name(w315) -> ("Waveforms"=w312:waveform(dbl)[], "RunCalculation.gain"=w313:dbl[])
            n105 = Divide(x=w312, y=w313) -> (x/y=w311:waveform(dbl)[])
            n106 = Bundle By Name(cluster=w315, "Waveforms"=w311) -> (w314:T12)
            n107 = call <vilib>:"Add State(s) to Queue__jki_lib_state_machine.vi"("State(s) in (\"\")"=w319) -> ("States Out"=w318:string)  [unwired: 14 in]
          }
          frame "DSP: Offset" {
            # "subtract any instrumental offsets"
            n108 = Unbundle By Name(w324) -> ("Waveforms"=w321:waveform(dbl)[], "RunCalculation.offset"=w322:dbl[])
            n109 = Subtract(x=w321, y=w322) -> (x-y=w320:waveform(dbl)[])
            n110 = Bundle By Name(cluster=w324, "Waveforms"=w320) -> (w323:T12)
            n111 = call <vilib>:"Add State(s) to Queue__jki_lib_state_machine.vi"("State(s) in (\"\")"=w328) -> ("States Out"=w327:string)  [unwired: 14 in]
          }
          frame "DSP: 60Hz Filter" {
            n112 = Unbundle By Name(w334) -> ("Waveforms"=w332:waveform(dbl)[])
            n113 = call "Prefilter_60Hz_Notch.vi"("error in (no error)"=w330, "Waveform In"=w332) -> ("error out"=w329:errorcluster, "Waveform Out"=w331:waveform(dbl)[])  [unwired: 8 in]
            n114 = Bundle By Name(cluster=w334, "Waveforms"=w331) -> (w333:T12)
            n115 = call <vilib>:"Add State(s) to Queue__jki_lib_state_machine.vi"("State(s) in (\"\")"=w337) -> ("States Out"=w336:string)  [unwired: 14 in]
          }
          frame "DSP: LP Filter" {
            n116 = Unbundle By Name(w344) -> ("Waveforms"=w342:waveform(dbl)[], "RunCalculation.LP config.high cutoff freq [Hz]"=w340:dbl)
            n117 = call "Prefilter_LP.vi"("error in (no error)"=w339, "high cutoff freq [Hz]"=w340, "Waveforms In"=w342) -> ("error out"=w338:errorcluster, "Waveforms Out"=w341:waveform(dbl)[])  [unwired: 7 in]
            n118 = Bundle By Name(cluster=w344, "Waveforms"=w341) -> (w343:T12)
            n119 = call <vilib>:"Add State(s) to Queue__jki_lib_state_machine.vi"("State(s) in (\"\")"=w347) -> ("States Out"=w346:string)  [unwired: 14 in]
          }
          frame "DSP: Lockin" {
            n120 = Unbundle By Name(w355) -> ("Self Reference"=w349:refnum<class "DSP.lvclass">, "RunCalculation.Lockin config"=w352:T5, "Waveforms"=w353:waveform(dbl)[])
            n121 = call "Lockin Engine.vi"("error in (no error)"=w354, "Signal in"=w353, "lockin config"=w352) -> ("error out"=w350:errorcluster, "Lockin Results"=w351:T17)  [unwired: 7 in]
            n122 = call "DSP.LockinResults.vi"("error in (no error)"=w350, "LockinResults"=w351, "DSP"=w349) -> ("error out"=w348:errorcluster)  [unwired: 7 in, 1 out]
            n123 = call <vilib>:"Add State(s) to Queue__jki_lib_state_machine.vi"("State(s) in (\"\")"=w358) -> ("States Out"=w357:string)  [unwired: 14 in]
          }
          frame "DSP: FFT" {
            # "decision trees queue other states"
            n124 = Unbundle By Name(w363) -> ("Waveforms"=w360:waveform(dbl)[], "RunCalculation.gain"=w361:dbl[])
            n125 = Divide(x=w360, y=w361) -> (x/y=w359:waveform(dbl)[])
            n126 = Bundle By Name(cluster=w363, "Waveforms"=w359) -> (w362:T12)
            n127 = call <vilib>:"Add State(s) to Queue__jki_lib_state_machine.vi"("State(s) in (\"\")"=w367) -> ("States Out"=w366:string)  [unwired: 14 in]
          }
        }
      }
    }
    frame Error {
    }
  }
  n128 = call-parent "Process.vi"("error in"=w7, "SMO"=w6) -> ("error out"=w4:errorcluster, "SMO out"=→"DSP out":refnum<class "DSP.lvclass">)  [unwired: 8 in]
  n129 = Merge Errors(w4, w3) -> (→"error out":errorcluster)
